vi "Module Not Running--error.vi"() -> (0 "error out":errorcluster)   [LabVIEW 2024, in "Scanner.lvlib"]
doc: "Outputs an error cluster containing a custom error code indicating the module is not running.\n_____\nBased on DQMH Dev Tools: Project Template 7.1.0.1503."
uses:
  Scanner.lvlib
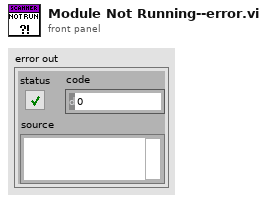
[diagram p1: front panel]
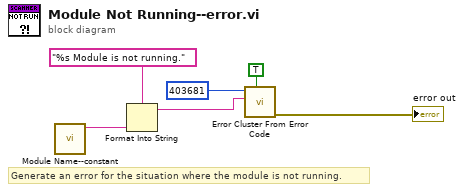
[diagram p0: block diagram]
diagram:
  # "Generate an error for the situation where the module is not running."
  n1 = call "Module Name--constant.vi"() -> ("Module Name"=w4:string)  [unwired: 11 in]
  n2 = Format Into String(format string="%s Module is not running.", w4) -> (resulting string=w2:string)  [unwired: 2 in, 1 out]
  n3 = call <vilib>:"Error Cluster From Error Code.vi"("show call chain? (False)"=TRUE, "error message (\"\")"=w2, "error code (0)"=403681) -> ("error out"=→"error out":errorcluster)  [unwired: 6 in]
